vi "VCI_CAN_OBJ_R.vi"() -> ()   [LabVIEW 2020]
panel:
  out "VCI_CAN_OBJ_R":T1={"ID"=0, "TimeStamp"=0, "TimeFlag"=0, "SendType"=1, "RemoteFlag"=0, "ExternFlag"=0, "DataLen"=8, "Data"=0, 0, 0, 0, 0, 0, 0, 0, "Reserved0"=0, "Reserved1"=0, "Reserved2"=0}
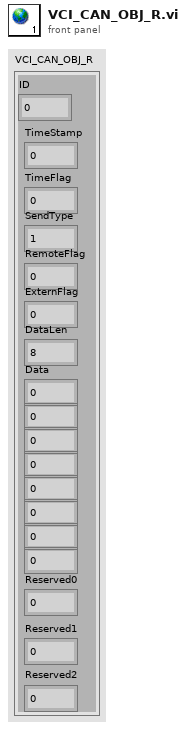
[diagram p1: front panel]
types:
  T1 = cluster{"ID":u32, "TimeStamp":u32, "TimeFlag":u8, "SendType":u8, "RemoteFlag":u8, "ExternFlag":u8, "DataLen":u8, "Data":u8, u8, u8, u8, u8, u8, u8, u8, "Reserved0":u8, "Reserved1":u8, "Reserved2":u8}
diagram:
